vi "DialogCloneLib.vi"(0 "LibWriter":refnum<class "LibWriter.lvclass">, 1 "ClassItemRefIn":refnum<vi>, 5 "error in (no error)":errorcluster) -> (14 "LibWriter":refnum<class "LibWriter.lvclass">, 15 "ClassItemRefOut":refnum<vi>, 16 "NewClassPath":path, 17 "Cancelled":bool, 19 "error out":errorcluster)   [LabVIEW 2014, in "LibWriter.lvclass"]
uses:
  <resource>/Framework/Providers/Open_GDS/ClassProviders/LibProvider_BaseClassInterface/LibWriter_class/ClassWriter_class/LibWriter.lvclass
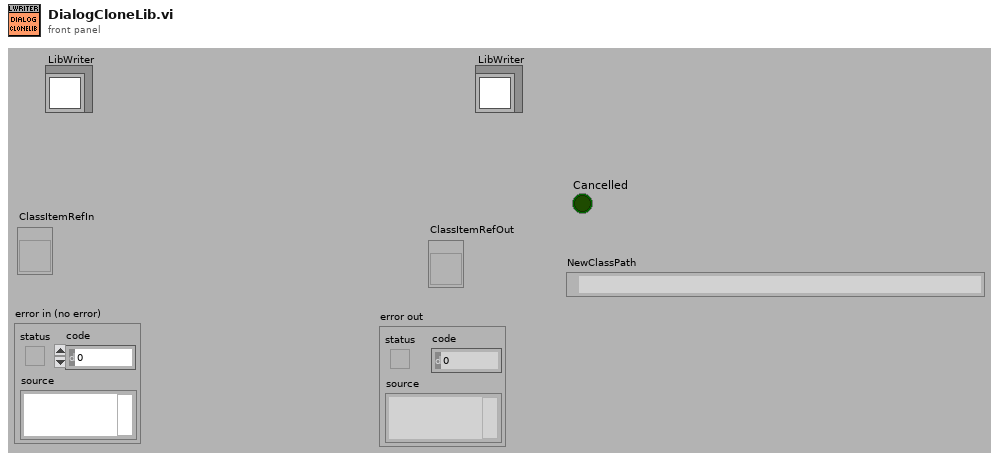
[diagram p1: front panel]
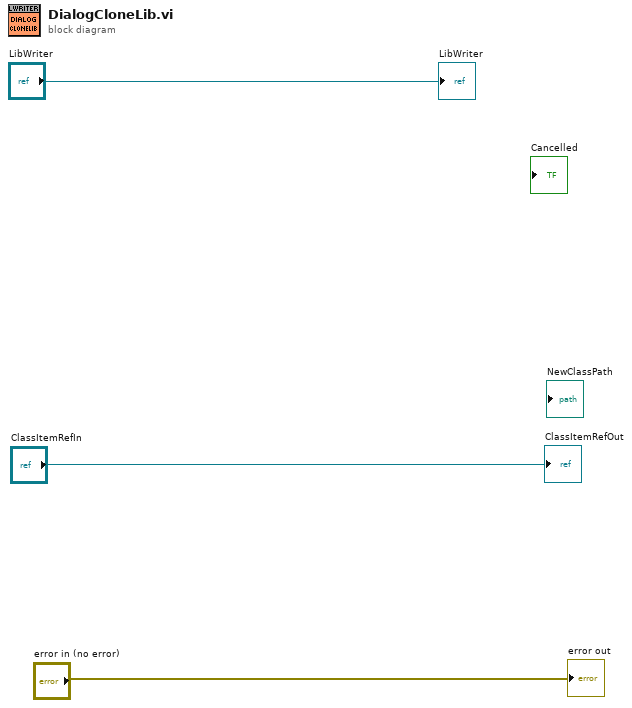
[diagram p0: block diagram]
diagram:
  "ClassItemRefOut" <- "ClassItemRefIn"
  "error out" <- "error in (no error)"
  "LibWriter" <- "LibWriter"
